vi "Rate Selective Filter Demonstrator.vi"() -> ()   [LabVIEW 2011]
uses:
  <vilib>/Utility/file.llb/Read From Spreadsheet File (DBL).vi
  <vilib>/Utility/file.llb/Write To Spreadsheet File (DBL).vi
panel:
  in  "Hyster":dbl=0.3
  in  "hi limit":dbl=50.0
  in  "lo limit":dbl
  out "num cols":i32
  out "num rows":i32
  out "Time":dbl
  out "Distance":dbl
  out "Mode":bool
  out "Waveform Chart":cluster{dbl, dbl}(graph)
  out "Filtered":dbl
  in  "Rate Thresh":dbl=25.0 step=0.001
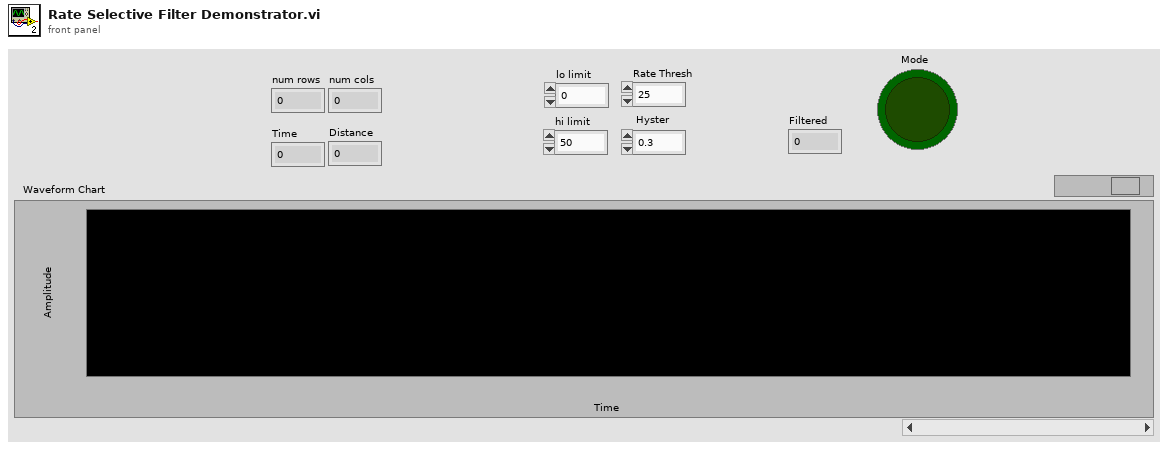
[diagram p1: front panel]
types:
  T1 = enum16{"open", "replace", "create", "open or create", "replace or create", "replace or create with confirmation"}
  T2 = cluster{dbl, dbl, dbl, dbl, "f":dbl, dbl, dbl, dbl, dbl, dbl, dbl}
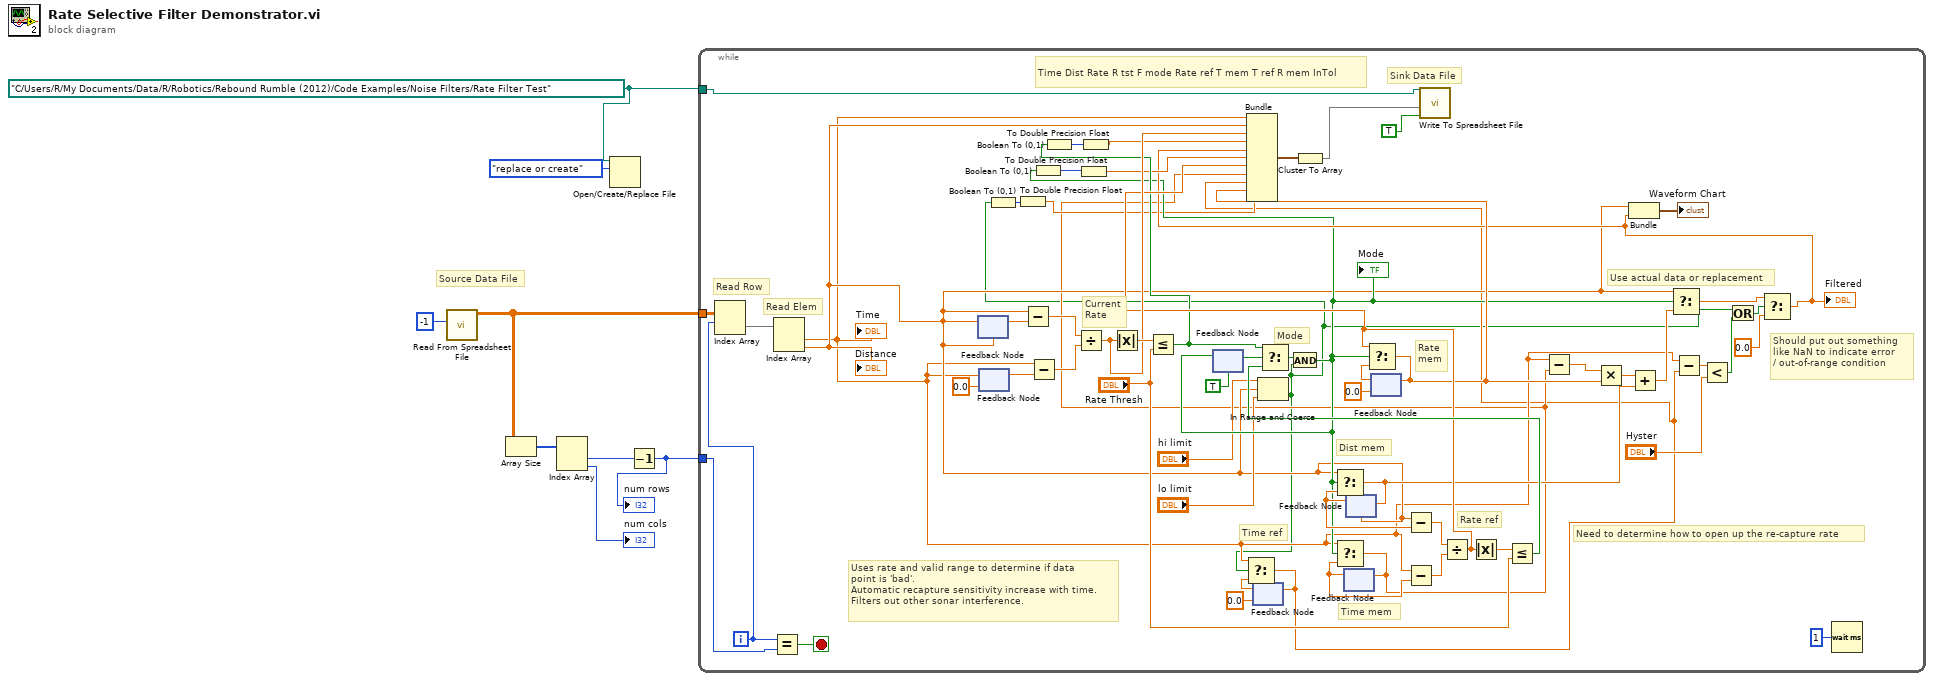
[diagram p0: block diagram]
diagram:
  w2 = path "C:/Users/R/My Documents/Data/R/Robotics/Rebound Rumble (2012)/Code Examples/Noise Filters/Rate Filter Test" ("datalog path (use dialog)")
  # "Source Data File"
  n1 = call-poly <vilib>:"Read From Spreadsheet File.vi"("number of rows (all:-1)"=-1) -> ("all rows"=w4:dbl[][])  [unwired: 6 in, 4 out]
  n2 = Array Size(array=w4) -> (size(s)=w7:i32[])
  n3 = Index Array(array=w7) -> (element #1=w5:i32, element #2=→"num cols":i32)  [unwired: 2 in]
  n4 = Open/Create/Replace File(file path (use dialog)=w2, operation (0:open)=T1."replace or create") -> ()  [unwired: 1 in, 6 out]
  n5 = Decrement(x=w5) -> (x-1=w3:i32)
  "num rows" <- w3
  n6 = while {
    tunnel: w4 -> [w46]
    tunnel: w3 -> [w44]
    tunnel: w2 -> [w43]
    i -> [w41]
    stop <- w45 stop-if-true
    # "Use actual data or replacement"
    # "Rate ref"
    # "Current\nRate"
    # "Time\tDist\tRate\tR tst\tF\tmode\tRate ref\tT mem\tT ref\tR mem\tInTol"
    # "Time ref"
    # "Sink Data File"
    # "Read Elem"
    # "Read Row"
    # "Uses rate and valid range to determine if data\npoint is 'bad'.\nAutomatic recapture sensitivity increase with time.\nFilters out other sonar interference."
    # "Need to determine how to open up the re-capture rate"
    # "Should put out something\nlike NaN to indicate error\n/ out-of-range condition"
    # "Rate\nmem"
    # "Mode"
    # "Time mem"
    # "Dist mem"
    n7 = Index Array(array=w46, index (row)=w41) -> (element=w47:dbl[])  [unwired: 1 in]
    n8 = Equal?(x=w41, y=w44) -> (x = y?=w45:bool)
    n9 = Index Array(array=w47) -> (element #1=w18:dbl, element #2=w24:dbl)  [unwired: 2 in]
    "Time" <- w18
    "Distance" <- w24
    n10 = feedback-in #1(w24) -> ()
    n11 = feedback #1(w24) -> (w64:dbl)
    n12 = feedback #2(0.0) -> (w63:dbl)
    n13 = feedback-in #2(w18) -> ()
    n14 = Subtract(x=w24, y=w64) -> (x-y=w68:dbl)
    n15 = Subtract(x=w18, y=w63) -> (x-y=w67:dbl)
    n16 = Divide(x=w68, y=w67) -> (x/y=w42:dbl)
    n17 = Absolute Value(x=w42) -> (abs(x)=w62:dbl)
    n18 = Less Or Equal?(x=w62, y="Rate Thresh") -> (x <= y?=w35:bool)
    n19 = Boolean To (0,1)(Boolean=w35) -> (0, 1=w34:i16)
    n20 = To Double Precision Float(number=w34) -> (double precision float=w33:dbl)
    n21 = feedback #3(TRUE) -> (w65:bool)
    n22 = feedback #4(0.0) -> (w21:dbl)
    n23 = In Range and Coerce(upper limit="hi limit", x=w24, lower limit="lo limit") -> (In Range?=w11:bool)  [unwired: 1 out]
    n24 = Boolean To (0,1)(Boolean=w11) -> (0, 1=w23:i16)
    n25 = To Double Precision Float(number=w23) -> (double precision float=w22:dbl)
    n26 = Select(t=w18, s=w11, f=w21) -> (s? t:f=w14:dbl)
    n27 = feedback-in #4(w14) -> ()
    n28 = feedback #5() -> (w58:dbl)  [unwired: 1 in]
    n29 = feedback #6(w24) -> (w59:dbl)
    n30 = feedback #7(0.0) -> (w54:dbl)
    n31 = Subtract(x=w24, y=w59) -> (x-y=w60:dbl)
    n32 = Subtract(x=w18, y=w58) -> (x-y=w61:dbl)
    n33 = Divide(x=w60, y=w61) -> (x/y=w38:dbl)
    n34 = Absolute Value(x=w38) -> (abs(x)=w57:dbl)
    n35 = Less Or Equal?(x=w57, y="Rate Thresh") -> (x <= y?=w55:bool)
    n36 = Select(t=w35, s=w65, f=w55) -> (s? t:f=w27:bool)
    n37 = And(x=w27, y=w11) -> (x .and. y?=w28:bool)
    "Mode" <- w28
    n38 = Boolean To (0,1)(Boolean=w28) -> (0, 1=w32:i16)
    n39 = To Double Precision Float(number=w32) -> (double precision float=w31:dbl)
    n40 = feedback-in #3(w28) -> ()
    n41 = Select(t=w24, s=w28, f=w59) -> (s? t:f=w37:dbl)
    n42 = Select(t=w18, s=w28, f=w58) -> (s? t:f=w15:dbl)
    n43 = feedback-in #5(w15) -> ()
    n44 = feedback-in #6(w37) -> ()
    n45 = Select(t=w38, s=w28, f=w54) -> (s? t:f=w36:dbl)
    n46 = feedback-in #7(w36) -> ()
    n47 = Subtract(x=w18, y=w15) -> (x-y=w53:dbl)
    n48 = Multiply(x=w53, y=w36) -> (x*y=w52:dbl)
    n49 = Add(x=w52, y=w37) -> (x+y=w51:dbl)
    n50 = Select(t=w24, s=w28, f=w51) -> (s? t:f=w19:dbl)
    n51 = Subtract(x=w18, y=w14) -> (x-y=w17:dbl)
    n52 = Less?(x=w17, y="Hyster") -> (x < y?=w10:bool)
    n53 = Or(x=w11, y=w10) -> (x .or. y?=w12:bool)
    n54 = Select(t=w19, s=w12, f=0.0) -> (s? t:f=w29:dbl)
    "Filtered" <- w29
    n55 = Bundle "Bundle"(w18, w24, w42, w33, "f"=w29, w31, w38, w15, w14, w36, w22) -> (w13:T2)  [unwired: 1 out]
    n56 = Cluster To Array(cluster=w13) -> (array=w39:dbl[])
    n57 = call-poly <vilib>:"Write To Spreadsheet File.vi"("append to file? (new file:F)"=TRUE, "1D data"=w39, "file path (dialog if empty)"=w43) -> ()  [unwired: 3 in, 3 out]
    n58 = Bundle(w24, "f"=w29) -> (→"Waveform Chart":cluster{dbl, "f":dbl})  [unwired: 1 in]
    n59 = Wait (ms)(milliseconds to wait=u32 1) -> ()  [unwired: 1 out]
  }
